vi "Dynamixel MX-Series Decode Bulk Pos Data FPGA.vi"(9 "ScaleOutput":fxp<+/-,25,16>=0.349609375, 11 "RecData":u8[](array[numeric])=[0, 0, 0, 0, 0, 0, 0, 0, 0, 0, 0, 0, 0, 0, 0, 0, 0, 0, 0, 0, 0, 0, 0, 0, 0, 0, 0, 0, 0, 0, 0, 0, 0, 0, 0, 0, 0, 0, 0, 0, 0, 0, 0, 0, 0, 0, 0, 0, 0, 0, 0, 0, 0, 0, 0, 0]) -> (0 "CError":bool, 1 "Checksum":u8[](array[numeric]), 3 "Position":fxp<+/-,24,16>[](array[numeric]) format="%.13g")   [LabVIEW 2015]
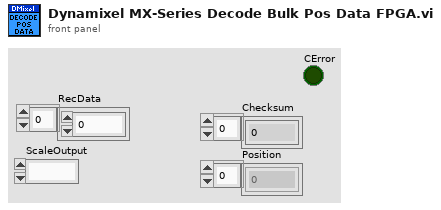
[diagram p1: front panel]
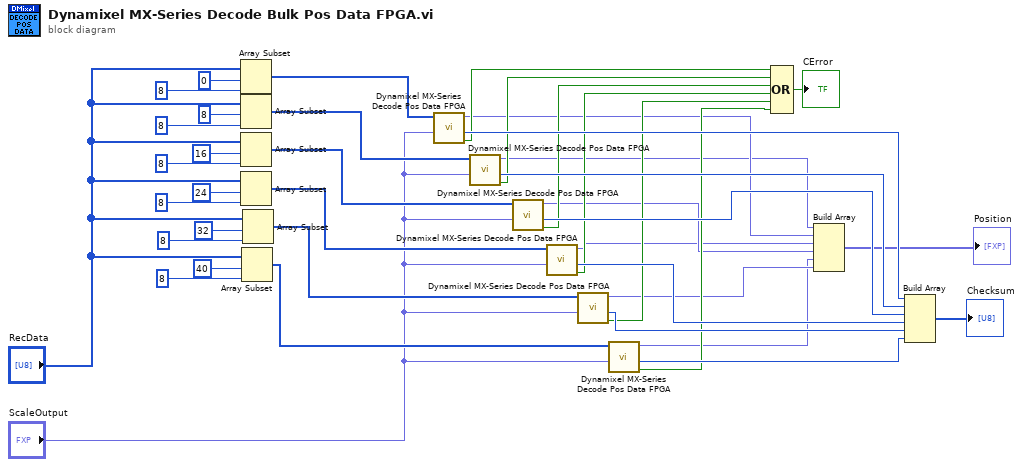
[diagram p0: block diagram]
diagram:
  n1 = Array Subset(array="RecData", index=0 ("length"), length=8) -> (w40:u8[])
  n2 = Array Subset(array="RecData", index=8 ("length"), length=8) -> (w27:u8[])
  n3 = Array Subset(array="RecData", index=16 ("length"), length=8) -> (w26:u8[])
  n4 = Array Subset(array="RecData", index=24 ("length"), length=8) -> (w25:u8[])
  n5 = Array Subset(array="RecData", index=40 ("length"), length=8) -> (w23:u8[])
  n6 = Array Subset(array="RecData", index=32 ("length"), length=8) -> (w24:u8[])
  n7 = call "Dynamixel MX-Series Decode Pos Data FPGA.vi"("ScaleOutput"="ScaleOutput", "RecData"=w40) -> ("Error"=w14:bool, "Csum"=w21:u8, "Position"=w7:fxp<+/-,24,16>)  [unwired: 7 in]
  n8 = call "Dynamixel MX-Series Decode Pos Data FPGA.vi"("ScaleOutput"="ScaleOutput", "RecData"=w27) -> ("Error"=w13:bool, "Csum"=w20:u8, "Position"=w6:fxp<+/-,24,16>)  [unwired: 7 in]
  n9 = call "Dynamixel MX-Series Decode Pos Data FPGA.vi"("ScaleOutput"="ScaleOutput", "RecData"=w26) -> ("Error"=w12:bool, "Csum"=w19:u8, "Position"=w5:fxp<+/-,24,16>)  [unwired: 7 in]
  n10 = call "Dynamixel MX-Series Decode Pos Data FPGA.vi"("ScaleOutput"="ScaleOutput", "RecData"=w25) -> ("Error"=w11:bool, "Csum"=w18:u8, "Position"=w4:fxp<+/-,24,16>)  [unwired: 7 in]
  n11 = call "Dynamixel MX-Series Decode Pos Data FPGA.vi"("ScaleOutput"="ScaleOutput", "RecData"=w24) -> ("Error"=w10:bool, "Csum"=w17:u8, "Position"=w3:fxp<+/-,24,16>)  [unwired: 7 in]
  n12 = call "Dynamixel MX-Series Decode Pos Data FPGA.vi"("ScaleOutput"="ScaleOutput", "RecData"=w23) -> ("Error"=w9:bool, "Csum"=w16:u8, "Position"=w2:fxp<+/-,24,16>)  [unwired: 7 in]
  n13 = Compound Arithmetic op=OR(w14, w13, w12, w11, w10, w9) -> (→"CError":bool)
  n14 = Build Array(w6, w7, w4, w5, w2, w3) -> (→"Position":fxp<+/-,24,16>[])
  n15 = Build Array(w21, w20, w19, w18, w17, w16) -> (→"Checksum":u8[])
